vi "Unflatten Value.vi"(8 "Error In":errorcluster, 10 "Value":string, 11 "2D String In":refnum<class "2D String.lvclass">) -> (0 "Error Out":errorcluster, 3 "2D String Out":refnum<class "2D String.lvclass">)   [LabVIEW 2020, in "NI_VIAnCFGDataStructure.lvlib" / "2D String.lvclass"]
doc: "Dynamic dispatch interface for unflattening Tree Data classes from string."
uses:
  <vilib>/addons/analyzer/VIAnCFGDataStructure/Data Types/2D String/2D String.lvclass
  <vilib>/addons/analyzer/VIAnCFGDataStructure/Data Types/2D String/2D String.lvclass/2D String.ctl
  <vilib>/addons/analyzer/VIAnCFGDataStructure/Tree Manager/API/Generate Hash.vi
  <vilib>/regexp/Match Regular Expression.xnode
  <vilib>/addons/analyzer/VIAnCFGDataStructure/Tree Manager/Tree.lvclass
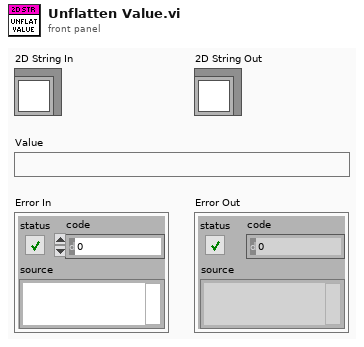
[diagram p1: front panel]
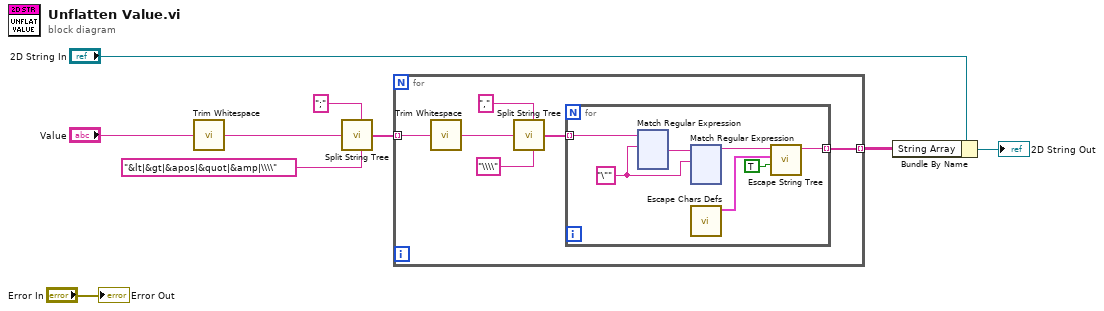
[diagram p0: block diagram]
diagram:
  n1 = call <vilib>:"Trim Whitespace.vi"("string"="Value") -> ("trimmed string"=w1:string)  [unwired: 1 in]
  n2 = call <vilib>:"Split String Tree.vi"("Ignore Pattern"="&lt|&gt|&apos|&quot|&amp|\\\\" ("Ignore Pattern  (\\)"), "Split Pattern"=";", "Input String"=w1) -> ("Split String"=w3:string[])  [unwired: 4 in]
  n3 = for {
    tunnel: w3 -> [w14] mode=indexing
    tunnel: [w13] -> w6 mode=indexing
    n4 = call <vilib>:"Trim Whitespace.vi"("string"=w14) -> ("trimmed string"=w10:string)  [unwired: 1 in]
    n5 = call <vilib>:"Split String Tree.vi"("Ignore Pattern"="\\\\", "Split Pattern"=",", "Input String"=w10) -> ("Split String"=w12:string[])  [unwired: 4 in]
    n6 = for {
      tunnel: w12 -> [w20] mode=indexing
      tunnel: [w21] -> w13 mode=indexing
      w18 = "\"" ("regular expression")
      n7 = xnode "Match Regular Expression"("input string"=w20, "regular expression"=w18) -> ("after match"=w19:string)  [unwired: 4 in, 4 out]
      n8 = xnode "Match Regular Expression"("input string"=w19, "regular expression"=w18) -> ("before match"=w17:string)  [unwired: 4 in, 4 out]
      n9 = call <vilib>:"Escape Chars Defs.vi"() -> ("Escapes"=w16:cluster{"String":string, "Escape":string}[])  [unwired: 11 in]
      n10 = call <vilib>:"Escape String Tree.vi"("Reverse? (False)"=TRUE ("Remove Escapes? (False)"), "Escapes"=w16, "String In"=w17) -> ("String Out"=w21:string)  [unwired: 8 in]
    }
  }
  n11 = Bundle By Name(cluster="2D String In", "String Array"=w6) -> (→"2D String Out":refnum<class "2D String.lvclass">)
  "Error Out" <- "Error In"
